vi "GetOperationOutput.vi"(8 "error in (no error)":errorcluster, 9 "Operation Output/Error In":string, 10 "Operation succeeded?":bool, 11 "Operation Name":string) -> (2 "Operation Output/Error Out":string, 3 "CLI Process Return Code":i32)   [LabVIEW 2014]
panel:
  in  "Format Error Output String":string="Error Code : %d\\nError Message : %s\\nAn error occurred while running the %s operation.\\n"
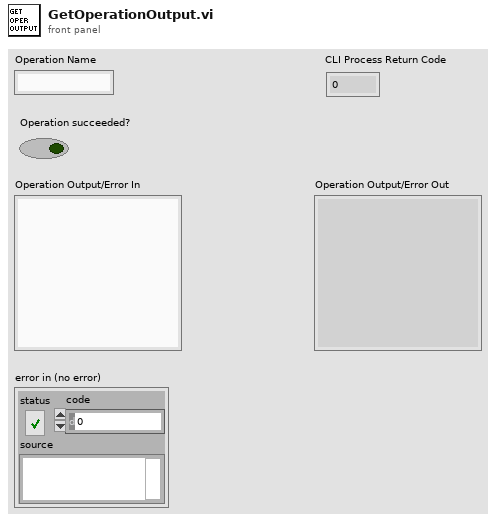
[diagram p1: front panel]
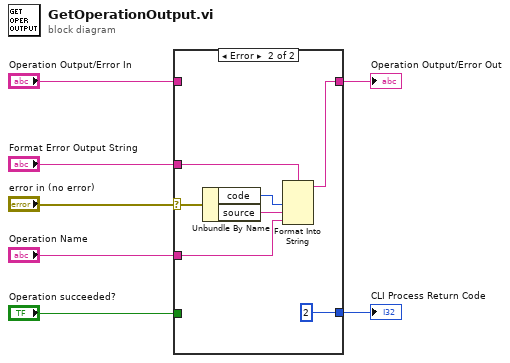
[diagram p0: block diagram]
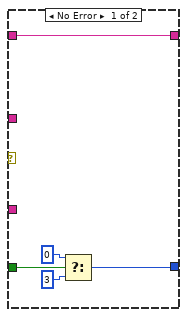
[diagram p2: hidden frame]
diagram:
  n1 = case shown="Error" "error in (no error)" {
    selector: "error in (no error)" -> [_ w16]
    tunnel: [w12 w13] -> w6
    tunnel: "Operation Output/Error In" -> [w12 _]
    tunnel: "Operation succeeded?" -> [w11 _]
    tunnel: [w10 2 ("f")] -> w3
    tunnel: "Format Error Output String" -> [_ w18]
    tunnel: "Operation Name" -> [_ w17]
    frame No Error {
      n2 = Select(t=0, s=w11, f=3) -> (s? t:f=w10:i32)
    }
    frame Error {
      n3 = Unbundle By Name(w16) -> ("code"=w15:i32, "source"=w14:string)
      n4 = Format Into String(format string=w18, w15, w14, w17) -> (resulting string=w13:string)  [unwired: 2 in, 1 out]
    }
  }
  "CLI Process Return Code" <- w3
  "Operation Output/Error Out" <- w6
